vi "16.1 Locate Pattern.vi"() -> ()   [LabVIEW 2016]
uses:
  <vilib>/vision/NI_Vision_Development_Module.lvlib
panel:
  out "Cap":T1(plugin-control)
  out "Image":T1(plugin-control)
  out "Coordinate System Out":T2 {"Measurement System"."Axis Reference" items=["Direct", "Indirect"]; "Measurement System"."Angle (deg)" format="%.2f"; "Measurement System"."Origin"."Y" format="%.2f"; "Measurement System"."Origin"."X" format="%.2f"; "Reference System"."Axis Reference" items=["Direct", "Indirect"]; "Reference System"."Angle (deg)" format="%.2f"; "Reference System"."Origin"."Y" format="%.2f"; "Reference System"."Origin"."X" format="%.2f"}
  # "Search bottle \ncap to set up\nmesurement \ncoordination\nsystem."
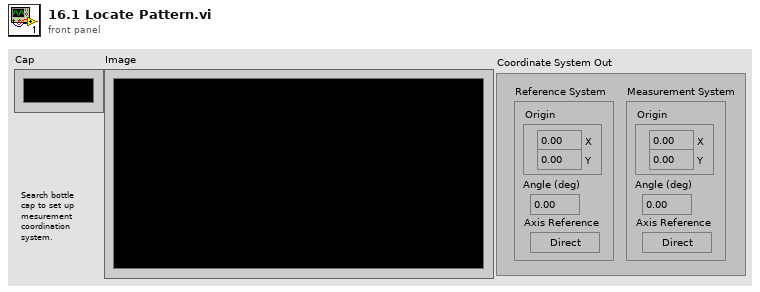
[diagram p1: front panel]
types:
  T1 = typedef "IMAQ Image.ctl" = refnum<image>
  T2 = typedef "IMAQ Coordinate System" = cluster{"Reference System":cluster{"Origin":cluster{"X":sgl, "Y":sgl}, "Angle (deg)":sgl, "Axis Reference":u32}, "Measurement System":cluster{"Origin":cluster{"X":sgl, "Y":sgl}, "Angle (deg)":sgl, "Axis Reference":u32}}
  T3 = cluster{"Algorithm":i32, "Minimum Match Score":sgl, "SubPixel Accuracy":bool, "Rotation Angle Ranges":cluster{"Start":sgl, "End":sgl}[], "Show Search Area":bool, "Show Feature Found":bool, "Show Result":bool}
  T4 = typedef "IMAQ Rectangle" = cluster{"Left":i32, "Top":i32, "Right":i32, "Bottom":i32, "Rotation":dbl}
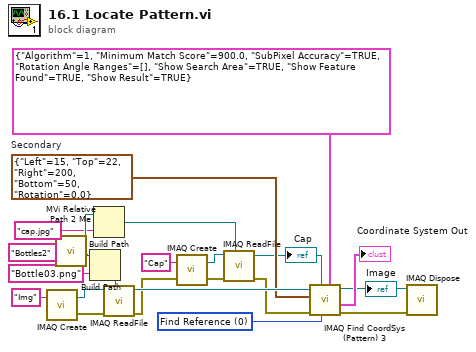
[diagram p0: block diagram]
diagram:
  w17 = u16 0 items=["Find Reference", "Update CoordSys"] ("Mode")
  w10 = T4 {"Left"=15, "Top"=22, "Right"=200, "Bottom"=50, "Rotation"=0.0}  # Secondary
  n1 = call "IMAQ Create"("Image Name"="Img") -> ("Src"=w20:T1, "error out"=w21:errorcluster)  [unwired: 4 in]
  n2 = call "MVi Relative Path 2 Me.vi"("Relative Path"="Bottles2" ("name or relative path")) -> ("Appended Dir"=w14:path)  [unwired: 5 in, 1 out]
  n3 = Build Path(base path=w14, name or relative path="Bottle03.png") -> (appended path=w15:path)
  n4 = Build Path(base path=w14, name or relative path="cap.jpg") -> (appended path=w12:path)
  n5 = call "IMAQ ReadFile"("File Path"=w15, "error in (no error)"=w21, "Image"=w20) -> ("error out"=w4:errorcluster, "Image Out"=w16:T1)  [unwired: 4 in, 3 out]
  n6 = call "IMAQ Create"("Image Name"="Cap", "error in (no error)"=w4) -> ("Src"=w2:T1, "error out"=w3:errorcluster)  [unwired: 3 in]
  n7 = call "IMAQ ReadFile"("File Path"=w12, "error in (no error)"=w3, "Image"=w2) -> ("error out"=w11:errorcluster, "Image Out"=w1:T1)  [unwired: 4 in, 3 out]
  "Cap" <- w1
  n8 = call "IMAQ Find CoordSys (Pattern) 3"("Settings"=T3 {"Algorithm"=1, "Minimum Match Score"=900.0, "SubPixel Accuracy"=TRUE, "Rotation Angle Ranges"=[], "Show Search Area"=TRUE, "Show Feature Found"=TRUE, "Show Result"=TRUE}, "Mode"=w17, "Template"=w1, "error in"=w11, "Search Rect"=w10, "Image"=w16) -> ("error out"=w9:errorcluster, "Coordinate System Out"=→"Coordinate System Out":T2, "Image Out"=w6:T1)  [unwired: 1 in, 2 out]
  "Image" <- w6
  n9 = call "IMAQ Dispose"("Image"=w6, "error in (no error)"=w9) -> ()  [unwired: 4 in, 1 out]
